vi "testMissingVi.vi"() -> ()   [LabVIEW 2020]
uses:
  node_type.ctl
  node.ctl
  terminalData.ctl
  terminal_type.ctl
  terminal_direction.ctl
  d2cbbd9a-39bd-4934-8608-8b79aaeda0e4.vi
  <vilib>/JDP Science/JSONtext/Variant to JSON Text.vi
  <vilib>/JDP Science/JSONtext/LVClass Serializer/JSONtext LVClass Serializer.lvclass
panel:
  in  "Debug":bool
  out "未处理类型":set{string}(c389)
  out "大小":i32
  in  "文件路径（使用对话框）":path=path "C:/Users/Fred/Desktop/LabAI/data/main.json"
  out "json_output":string
  out "分析时间":dbl format="%.3f s"
  in  "Path to Entrance VI":path=path "C:/Users/Fred/Desktop/LabAI/mainV2.vi"
  # "C:\\Users\\Fred\\Desktop\\FL62风洞主控软件\\Desktop\\2.4米风洞主控软件20240716\\主程序 - 一键启动-web.vi"
  # "C:\\Users\\Fred\\Desktop\\LabAI\\mainV2.vi"
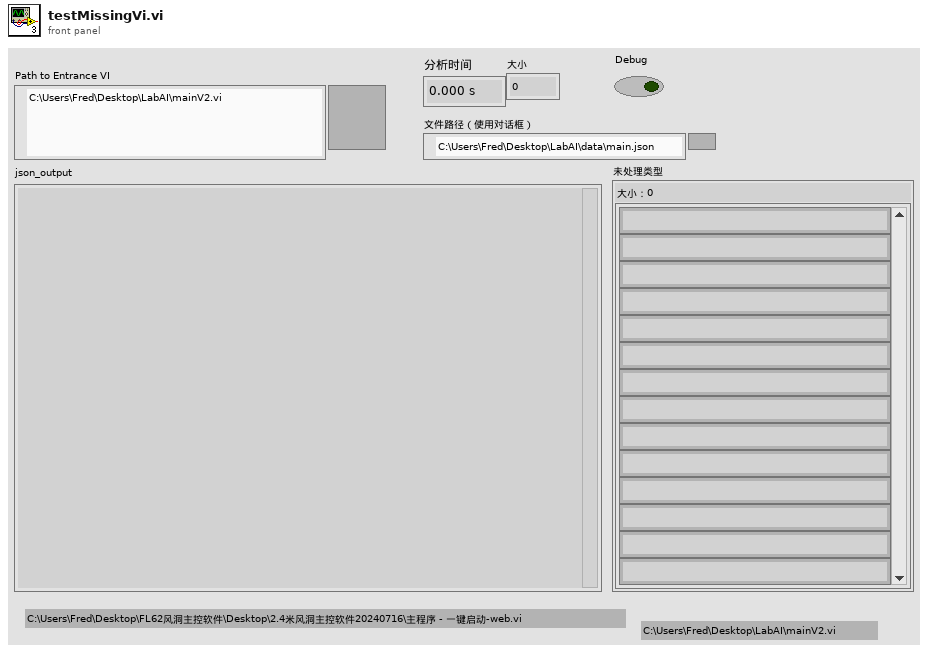
[diagram p1: front panel]
types:
  T1 = typedef "node.ctl" = cluster{"id":string, "name":string, "VIName":string, "VIPath":string, "type":string, "label":string, "parentId":string, "nodes":variant[], "frames":variant[], "properties":variant[], "metadata":variant[], "terminals":T2[]}
  T2 = typedef "terminalData.ctl" = cluster{"ThisUID":i32, "ThisName":string, "type":T3, "direction":T4, "datatype":string, "EndTerminalUID":i32, "EndTerminaltName":string, "EndGobjectUID":i32, "EndObjectClass":string}
  T3 = typedef "terminal_type.ctl" = enum16{"selector", "tunnel", "shift", "timeout", "normal", "floating"}
  T4 = typedef "terminal_direction.ctl" = enum16{"input", "output"}
  T5 = typedef "node_type.ctl" = enum16{"VI", "SubVI", "Function", "ForLoop", "WhileLoop", "Frame", "CaseStructure", "EventStructure"}
  T6 = enum16{"open", "replace", "create", "open or create", "replace or create", "replace or create with confirmation"}
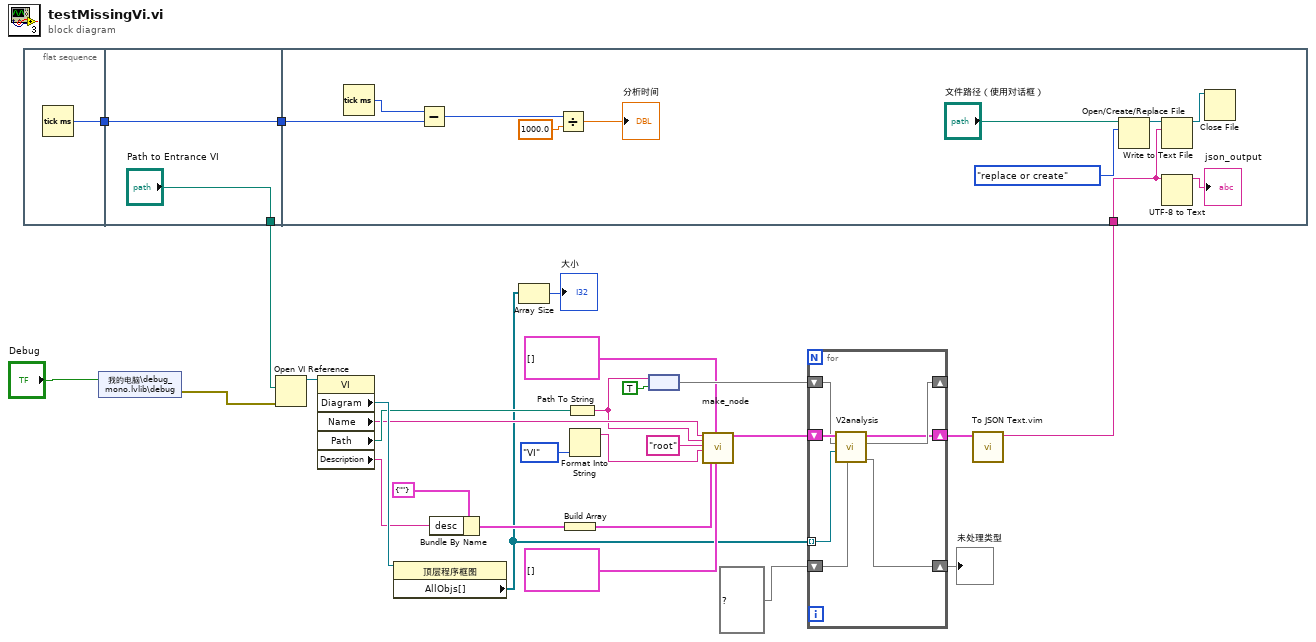
[diagram p0: block diagram]
diagram:
  n1 = flat-sequence {
    tunnel: [w29] -> w28
    tunnel: ["Path to Entrance VI"] -> w23
    tunnel: w28 -> [w30]
    tunnel: [w30] -> w27
    tunnel: w27 -> [w41]
    tunnel: w12 -> [w33]
    frame #0 {
      n2 = Tick Count (ms) ("时间计数器")() -> (millisecond timer value=w29:u32)
    }
    frame #1 {
    }
    frame #2 {
      n3 = Tick Count (ms) ("时间计数器")() -> (millisecond timer value=w42:u32)
      n4 = Subtract ("减")(x=w42, y=w41) -> (x-y=w39:u32)
      n5 = Divide ("除")(x=w39, y=1000.0) -> (x/y=→"分析时间":dbl)
      n6 = Open/Create/Replace File ("打开/创建/替换文件")(file path (use dialog)="文件路径（使用对话框）", operation (0:open)=T6."replace or create" ("操作(0:open)")) -> (refnum out=w35:refnum<file>)  [unwired: 4 in, 2 out]
      n7 = Write to Text File ("写入文本文件")(file (use dialog)=w35, text=w33) -> (refnum out=w34:refnum<file>)  [unwired: 2 in, 2 out]
      n8 = UTF-8 to Text ("UTF-8至文本转换")(11:w33) -> (3:→"json_output":string)  [unwired: 2 in, 1 out]
      n9 = Close File ("关闭文件")(refnum=w34) -> ()  [unwired: 1 in, 2 out]
    }
  }
  n10 = shared-variable "我的电脑\\debug_mono.lvlib\\debug"("Debug") -> (error out=w1:errorcluster)  [unwired: 1 in]
  n11 = Open VI Reference ("打开VI引用")(vi path=w23, error in (no error)=w1) -> (vi reference=w26:refnum<vi>)  [unwired: 4 in, 1 out]
  n12 = property on="属性节点" class="VI"(reference=w26) -> ("Diagram"=w25:refnum<vi>, "Name"=w22:string, "Path"=w24:path, "Description"=w8:string)  [unwired: 1 in, 2 out]
  n13 = property on="属性节点" class="顶层程序框图"(reference=w25) -> ("AllObjs[]"=w6:refnum<vi>[])  [unwired: 1 in, 2 out]
  n14 = Bundle By Name ("按名称捆绑")(cluster=cluster{"desc":string} {"desc"=""}, "desc"=w8) -> (w9:cluster{"desc":string})
  n15 = Array Size ("数组大小")(array=w6) -> (size(s)=→"大小":i32)
  n16 = Build Array ("创建数组")(w9) -> (w7:cluster{"desc":string}[])
  n17 = Path To String ("路径至字符串转换")(path=w24) -> (string=w16:string)
  n18 = Format Into String ("格式化写入字符串")(node_type."VI" ("枚举")) -> (resulting string=w19:string)  [unwired: 3 in, 1 out]
  n19 = node ("生成映射表")(w16, TRUE) -> (w14:map{string, bool})
  n20 = call "make_node.vi"("VIName"=w22, "VIPath"=w16, "id"="root", "type"=w19, "metadata"=w7, "frames"=T1[] [] ("nodes"), "nodes"=T1[] []) -> ("node"=w17:T1)  [unwired: 12 in]
  n21 = for {
    tunnel: w6 -> [w49] mode=indexing
    shift-right: [w46] -> _
    shift-left: w14 -> [w47]
    shift-right: [w45] -> w13
    shift-left: w17 -> [w48]
    shift-right: [w43] -> w4
    shift-left: set{string} {} ("set") -> [w44]
    n22 = call "V2analysis.vi"("node_in"=w48, "VIPathMap"=w47, "GObj引用句柄"=w49, "集合"=w44) -> ("node_out"=w45:T1, "VIPathMap 2"=w46:map{string, bool}, "集合 2"=w43:set{string})  [unwired: 4 in]
  }
  "未处理类型" <- w4
  n23 = call "To JSON Text.vim"("Anything"=w13) -> ("<JSON>"=w12:string)  [unwired: 9 in, 1 out]
